vi "config dual Spark Max.vi"(11 "motor\ndefaults":T1[](array[typedef]) {"gear ratio" format="%_5f"; "MOTOR SELECT" items=["REV NEO"=5676, "REV NEO 550"=11000, "VEX Falcon"=6380, "WC Kraken"=6000]}) -> (0 "error out":errorcluster, 3 "MotorControlDevRef":T7)   [LabVIEW 2023]
uses:
  <vilib>/Rock Robotics/WPI/MotorControl/WPI_MotorControlDeviceRef.ctl
  <vilib>/Rock Robotics/WPI/MotorControl/WPI_MotorControlType.ctl
  <vilib>/Rock Robotics/SystemInterfaces/DIO/FPGA_DIOPWMChannel.ctl
  <vilib>/Rock Robotics/WPI/PWM/WPI_PWMDeadband.ctl
  <vilib>/Rock Robotics/SystemInterfaces/DIO/FPGA_DIOChannel.ctl
  ctrl defs/ctrl swerve motor.ctl
  ctrl defs/ctrl MOTOR SELECT.ctl
  <vilib>/Rock Robotics/WPI/ThirdParty/REV Robotics/REVLib/Typedef/Spark MAX Idle Mode.ctl
  ctrl defs/ctrl Spark MAX current limiting.ctl
  ctrl defs/ctrl motor PIDF coefficients.ctl
  <vilib>/Rock Robotics/WPI/ThirdParty/REV Robotics/REVLib/Typedef/Spark MAX Smart Motion Parameters.ctl
  <vilib>/Rock Robotics/WPI/ThirdParty/REV Robotics/REVLib/Typedef/Spark MAX Motor Type.ctl
  <vilib>/Rock Robotics/WPI/ThirdParty/REV Robotics/REVLib/Typedef/Spark MAX Limit Switch Polarity.ctl
  <vilib>/Rock Robotics/WPI/ThirdParty/REV Robotics/REVLib/Typedef/Spark MAX Limit Direction.ctl
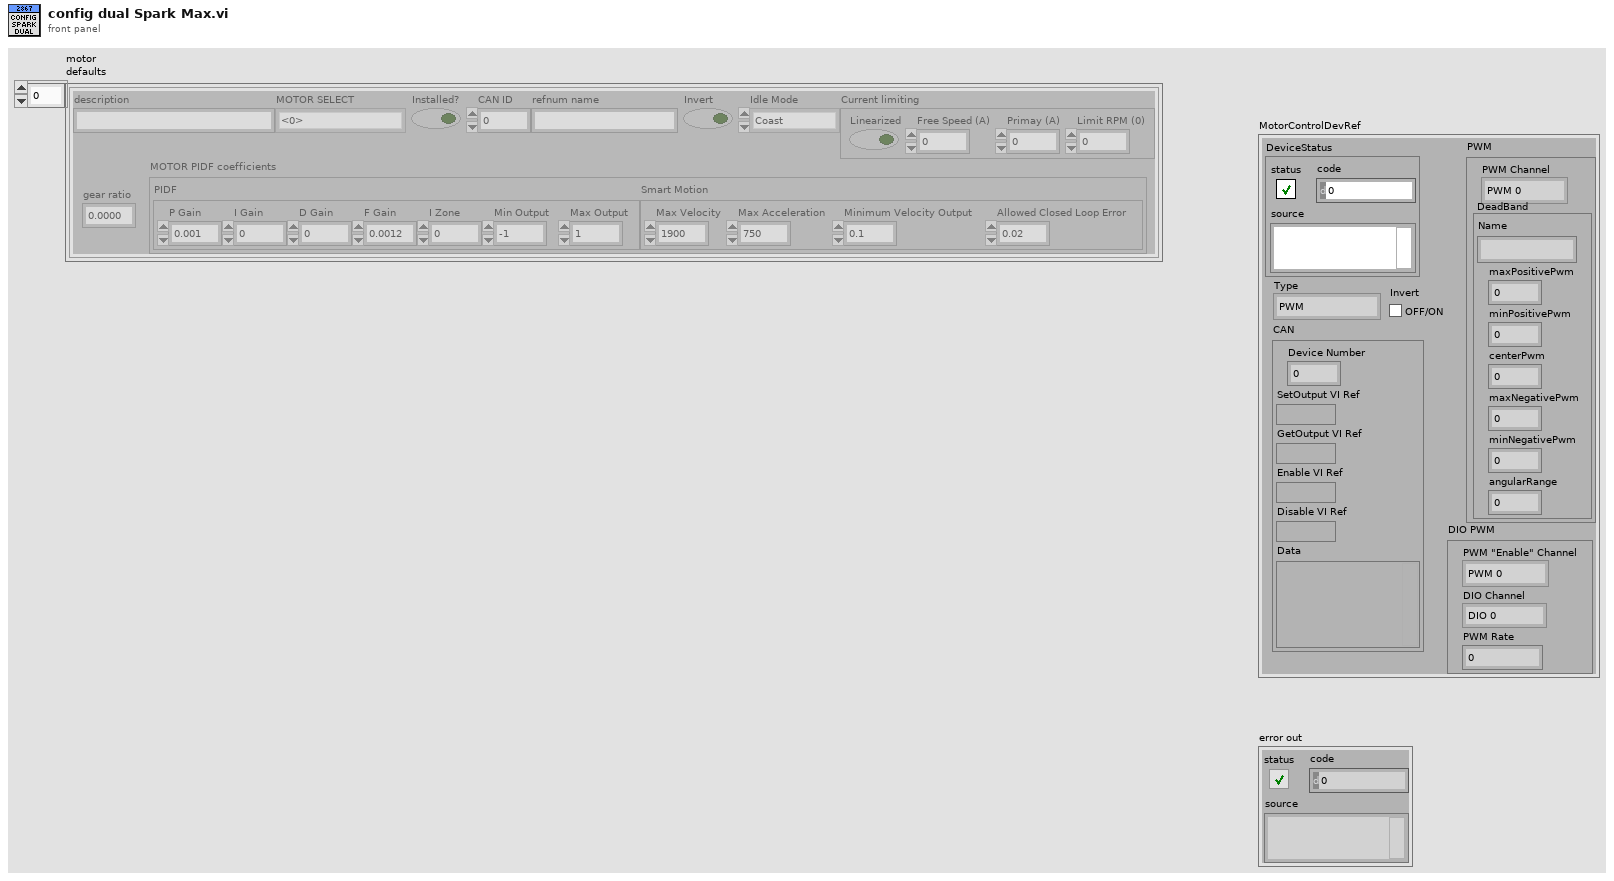
[diagram p1: front panel]
types:
  T1 = typedef "ctrl swerve motor.ctl" = cluster{"description":string, "MOTOR SELECT":T2, "Installed?":bool, "CAN ID":u8, "refnum name":string, "Invert":bool, "Idle Mode":T3, "Current limiting":T4, "MOTOR PIDF coefficients":T5, "gear ratio":dbl}
  T2 = typedef "ctrl MOTOR SELECT.ctl" = i16
  T3 = typedef "Spark MAX Idle Mode.ctl" = enum16{"Coast", "Brake"}
  T4 = typedef "ctrl Spark MAX current limiting.ctl" = cluster{"Linearized":bool, "Free Speed (A)":dbl, "Primay (A)":dbl, "Limit RPM (0)":u32}
  T5 = typedef "ctrl motor PIDF coefficients.ctl" = cluster{"PIDF":cluster{"P Gain":dbl, "I Gain":dbl, "D Gain":dbl, "F Gain":dbl, "I Zone":dbl, "Min Output":dbl, "Max Output":dbl}, "Smart Motion":T6}
  T6 = typedef "Spark MAX Smart Motion Parameters.ctl" = cluster{"Max Velocity":dbl, "Max Acceleration":dbl, "Minimum Velocity Output":dbl, "Allowed Closed Loop Error":dbl}
  T7 = typedef "WPI_MotorControlDeviceRef.ctl" = cluster{"DeviceStatus":errorcluster, "Type":T8, "PWM":cluster{"PWM Channel":T9, "DeadBand":T10}, "CAN":cluster{"Device Number":u8, "SetOutput VI Ref":variant, "GetOutput VI Ref":variant, "Enable VI Ref":variant, "Disable VI Ref":variant, "Data":variant}, "Invert":bool, "DIO PWM":cluster{"PWM \"Enable\" Channel":T9, "DIOChannel":T11, "PWM Rate":dbl}}
  T8 = typedef "WPI_MotorControlType.ctl" = enum16{"PWM", "CAN", "DIO PWM"}
  T9 = typedef "FPGA_DIOPWMChannel.ctl" = enum8{"PWM 0", "PWM 1", "PWM 2", "PWM 3", "PWM 4", "PWM 5", "PWM 6", "PWM 7", "PWM 8", "PWM 9", "PWM MXP 0", "PWM MXP 1", "PWM MXP 2", "PWM MXP 3", "PWM MXP 4", "PWM MXP 5", "PWM MXP 6", "PWM MXP 7", "PWM MXP 8", "PWM MXP 9", "Invalid"}
  T10 = typedef "WPI_PWMDeadband.ctl" = cluster{"Name":string, "maxPositivePwm":i32, "minPositivePwm":i32, "centerPwm":i32, "maxNegativePwm":i32, "minNegativePwm":i32, "angularRange":u16}
  T11 = typedef "FPGA_DIOChannel.ctl" = enum8{"DIO 0", "DIO 1", "DIO 2", "DIO 3", "DIO 4", "DIO 5", "DIO 6", "DIO 7", "DIO 8", "DIO 9", "DIO MXP 0", "DIO MXP 1", "DIO MXP 2", "DIO MXP 3", "DIO MXP 4", "DIO MXP 5", "DIO MXP 6", "DIO MXP 7", "DIO MXP 8", "DIO MXP 9", "DIO MXP 10", "DIO MXP 11", "DIO MXP 12", "DIO MXP 13", "DIO MXP 14", "DIO MXP 15", "SPI Port CS1", "SPI Port CS2", "SPI Port CS3", "SPI Port MISO", "SPI Port MOSI", "Invalid"}
  T12 = typedef "Spark MAX Motor Type.ctl" = enum16{"Brushed", "Brushless"}
  T13 = typedef "Spark MAX Limit Direction.ctl" = enum16{"Forward Limit", "Reverse Limit"}
  T14 = typedef "Spark MAX Limit Switch Polarity.ctl" = enum16{"Normally Open", "Normally Closed"}
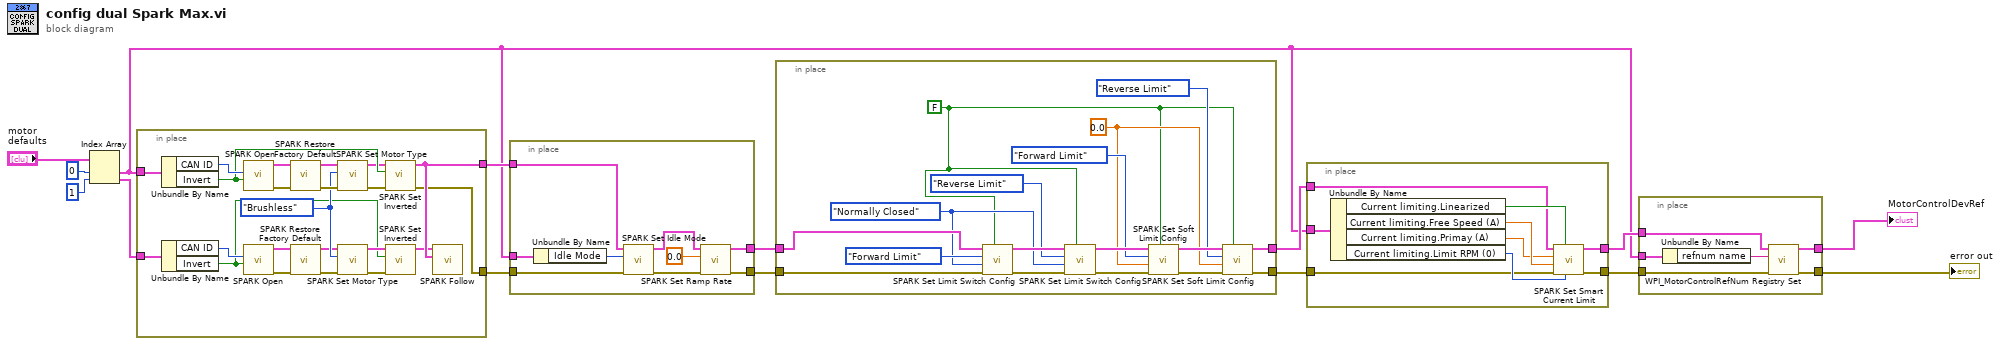
[diagram p0: block diagram]
diagram:
  n1 = Index Array(array="motor\ndefaults", index #1=0 ("index"), index #2=1 ("index")) -> (element #1=w4:T1, element #2=w1:T1)
  n2 = in-place {
    in-place-border: [w25] -> w11
    in-place-border: [w26] -> w10
    in-place-border: w4 -> [w32]
    in-place-border: w1 -> [w28]
    w27 = Spark_MAX_Motor_Type."Brushless" ("Motor Type")
    n3 = Unbundle By Name(w32) -> ("CAN ID"=w37:u8, "Invert"=w36:bool)
    n4 = Unbundle By Name(w28) -> ("CAN ID"=w24:u8, "Invert"=w17:bool)
    n5 = call <vilib>:"SPARK Open.vi"("Invert"=w36, "Device Number"=w37) -> ("error out"=w33:errorcluster, "MotorControlDeviceRef"=w34:T7)  [unwired: 8 in]
    n6 = call <vilib>:"SPARK Open.vi"("Invert"=w17, "Device Number"=w24) -> ("error out"=w21:errorcluster, "MotorControlDeviceRef"=w22:T7)  [unwired: 8 in]
    n7 = call <vilib>:"SPARK Restore Factory Default.vi"("error in"=w33, "MotorControlDeviceRef"=w34) -> ("error out"=w30:errorcluster, "MotorControlDeviceRef"=w35:T7)  [unwired: 8 in]
    n8 = call <vilib>:"SPARK Restore Factory Default.vi"("error in"=w21, "MotorControlDeviceRef"=w22) -> ("error out"=w19:errorcluster, "MotorControlDeviceRef"=w23:T7)  [unwired: 8 in]
    n9 = call <vilib>:"SPARK Set Motor Type.vi"("error in (no error)"=w30, "Motor Type"=w27, "MotorControlDevRef"=w35) -> ("error out"=w29:errorcluster, "MotorControlDeviceRef"=w31:T7)  [unwired: 7 in]
    n10 = call <vilib>:"SPARK Set Motor Type.vi"("error in (no error)"=w19, "Motor Type"=w27, "MotorControlDevRef"=w23) -> ("error out"=w18:errorcluster, "MotorControlDeviceRef"=w20:T7)  [unwired: 7 in]
    n11 = call <vilib>:"SPARK Set Inverted.vi"("error in (no error)"=w29, "Inverted (F)"=w36, "MotorControlDeviceRef in"=w31) -> ("error out"=w25:errorcluster, "MotorControlDeviceRef out"=w26:T7)  [unwired: 7 in]
    n12 = call <vilib>:"SPARK Set Inverted.vi"("error in (no error)"=w18, "Inverted (F)"=w17, "MotorControlDeviceRef in"=w20) -> ("MotorControlDeviceRef out"=w16:T7)  [unwired: 7 in, 1 out]
    n13 = call <vilib>:"SPARK Follow.vi"("Master Controller"=w26, "MotorControlDeviceRef"=w16) -> ()  [unwired: 8 in, 2 out]
  }
  n14 = in-place {
    in-place-border: w11 -> [w46]
    in-place-border: w10 -> [w45]
    in-place-border: [w41] -> w9
    in-place-border: [w39] -> w6
    in-place-border: w4 -> [w42]
    n15 = Unbundle By Name(w42) -> ("Idle Mode"=w43:T3)
    n16 = call <vilib>:"SPARK Set Idle Mode.vi"("error in (no error)"=w46, "Idle Mode"=w43, "MotorControlDeviceRef in"=w45) -> ("error out"=w40:errorcluster, "MotorControlDeviceRef out"=w44:T7)  [unwired: 7 in]
    n17 = call <vilib>:"SPARK Set Ramp Rate.vi"("error in (no error)"=w40, "Seconds from neutral to full (0)"=sgl 0.0, "MotorControlDeviceRef in"=w44) -> ("error out"=w39:errorcluster, "MotorControlDeviceRef"=w41:T7)  [unwired: 7 in]
  }
  n18 = in-place {
    in-place-border: w9 -> [w63]
    in-place-border: [w53] -> w7
    in-place-border: w6 -> [w57]
    in-place-border: [w47] -> w5
    w51 = 0.0 ("Soft Limit (0)")
    w58 = Spark_MAX_Limit_Switch_Polarity."Normally Closed" ("Polarity (Normally Open)")
    w50 = FALSE ("Enabled? (T)")
    n19 = call <vilib>:"SPARK Set Limit Switch Config.vi"("Enabled? (T)"=w50, "error in (no error)"=w57, "Polarity (Normally Open)"=w58, "Limit Switch"=Spark_MAX_Limit_Direction."Forward Limit", "MotorControlDeviceRef in"=w63) -> ("error out"=w56:errorcluster, "MotorControlDeviceRef out"=w62:T7)  [unwired: 5 in]
    n20 = call <vilib>:"SPARK Set Limit Switch Config.vi"("Enabled? (T)"=w50, "error in (no error)"=w56, "Polarity (Normally Open)"=w58, "Limit Switch"=Spark_MAX_Limit_Direction."Reverse Limit", "MotorControlDeviceRef in"=w62) -> ("error out"=w49:errorcluster, "MotorControlDeviceRef out"=w60:T7)  [unwired: 5 in]
    n21 = call <vilib>:"SPARK Set Soft Limit Config.vi"("Enabled? (T)"=w50, "error in (no error)"=w49, "Soft Limit (0)"=w51, "Soft Limit Switch"=Spark_MAX_Limit_Direction."Forward Limit", "MotorControlDeviceRef in"=w60) -> ("error out"=w48:errorcluster, "MotorControlDeviceRef out"=w55:T7)  [unwired: 5 in]
    n22 = call <vilib>:"SPARK Set Soft Limit Config.vi"("Enabled? (T)"=w50, "error in (no error)"=w48, "Soft Limit (0)"=w51, "Soft Limit Switch"=Spark_MAX_Limit_Direction."Reverse Limit", "MotorControlDeviceRef in"=w55) -> ("error out"=w47:errorcluster, "MotorControlDeviceRef out"=w53:T7)  [unwired: 5 in]
  }
  n23 = in-place {
    in-place-border: [w72] -> w14
    in-place-border: [w67] -> w12
    in-place-border: w7 -> [w66]
    in-place-border: w5 -> [w65]
    in-place-border: w4 -> [w64]
    n24 = Unbundle By Name(w64) -> ("Current limiting.Linearized"=w68:bool, "Current limiting.Free Speed (A)"=w70:dbl, "Current limiting.Primay (A)"=w69:dbl, "Current limiting.Limit RPM (0)"=w71:u32)
    n25 = call <vilib>:"SPARK Set Smart Current Limit.vi"("Linear Limit RPM (0)"=w71, "Linearized Limit Enabled (F)"=w68, "error in (no error)"=w65, "Free Speed Current Limit (20A)"=w70, "Primay Current Limit (80A)"=w69, "MotorControlDeviceRef in"=w66) -> ("error out"=w72:errorcluster, "MotorControlDeviceRef out"=w67:T7)  [unwired: 4 in]
  }
  n26 = in-place {
    in-place-border: [w78] -> w15
    in-place-border: w14 -> [w77]
    in-place-border: [w76] -> w13
    in-place-border: w12 -> [w75]
    in-place-border: w4 -> [w73]
    n27 = Unbundle By Name(w73) -> ("refnum name"=w74:string)
    n28 = call <vilib>:"WPI_MotorControlRefNum Registry Set.vi"("error in (no error)"=w77, "refnum name"=w74, "MotorControlDevRef"=w75) -> ("error out"=w78:errorcluster, "MotorControlDevRef"=w76:T7)  [unwired: 7 in]
  }
  "error out" <- w15
  "MotorControlDevRef" <- w13
